vi "formulaNodeEquiv.vi"() -> ()   [LabVIEW 2014]
panel:
  out "Conditional Function":cluster{"yValues":dbl[], "xValues":dbl[]}(graph)
  out "Sum Of Y Values":dbl(knob) scale=0.0..200.0
  in  "Step Size":dbl(knob)=3.0 scale=0.0..10.0
  in  "Frequency":dbl(knob)=0.3 scale=0.0..1.0
  in  "Amplitude":dbl(knob)=3.0 scale=0.0..10.0
  in  "Number of Elements":i32(knob)=50 scale=0.0..100.0
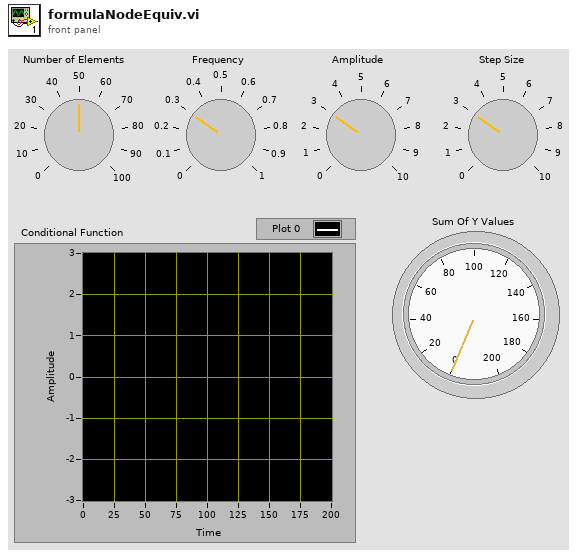
[diagram p1: front panel]
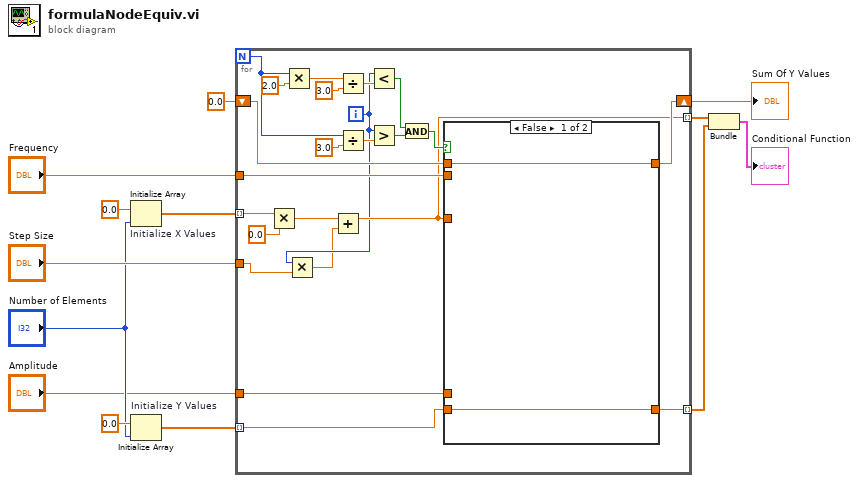
[diagram p0: block diagram]
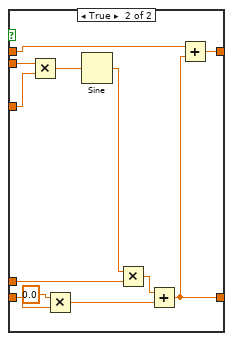
[diagram p2: hidden frame]
diagram:
  n1 = Initialize Array "Initialize X Values"(0.0 ("element"), "Number of Elements") -> (w11:dbl[])
  n2 = Initialize Array "Initialize Y Values"(0.0 ("element"), "Number of Elements") -> (w10:dbl[])
  n3 = for {
    N -> [w31]
    tunnel: w11 -> [w36] mode=indexing
    tunnel: w10 -> [w25] mode=indexing
    tunnel: "Amplitude" -> [w21]
    tunnel: "Frequency" -> [w23]
    tunnel: "Step Size" -> [w15]
    tunnel: [w17] -> w9 mode=indexing
    tunnel: [w24] -> w8 mode=indexing
    shift-right: [w19] -> w2
    shift-left: 0.0 -> [w20]
    i -> [w16]
    n4 = Multiply(x=w36, y=0.0) -> (x*y=w22:dbl)
    n5 = Multiply(x=w31, y=2.0) -> (x*y=w34:dbl)
    n6 = Multiply(x=w16, y=w15) -> (x*y=w14:dbl)
    n7 = Add(x=w22, y=w14) -> (x+y=w17:dbl)
    n8 = Divide(x=w34, y=3.0) -> (x/y=w29:dbl)
    n9 = Divide(x=w31, y=3.0) -> (x/y=w30:dbl)
    n10 = Less?(x=w16, y=w29) -> (x < y?=w27:bool)
    n11 = Greater?(x=w16, y=w30) -> (0:w28:bool)
    n12 = And(x=w27, y=w28) -> (x .and. y?=w26:bool)
    n13 = case shown="False" w26 {
      tunnel: w25 -> [w38 w50]
      tunnel: [w38 w40] -> w24
      tunnel: w23 -> [_ w46]
      tunnel: w17 -> [_ w45]
      tunnel: w21 -> [_ w43]
      tunnel: w20 -> [w37 w41]
      tunnel: [w37 w39] -> w19
      frame False {
      }
      frame True {
        n14 = Multiply(x=w46, y=w45) -> (x*y=w47:dbl)
        n15 = Multiply(x=0.0, y=w50) -> (x*y=w48:dbl)
        n16 = Sine(x=w47) -> (sin(x)=w44:dbl)
        n17 = Multiply(x=w44, y=w43) -> (x*y=w42:dbl)
        n18 = Add(x=w42, y=w48) -> (x+y=w40:dbl)
        n19 = Add(x=w41, y=w40) -> (x+y=w39:dbl)
      }
    }
  }
  "Sum Of Y Values" <- w2
  n20 = Bundle(w9, w8) -> (→"Conditional Function":cluster{dbl[], dbl[]})  [unwired: 1 in]
